vi "Get ROI Statistics String.vi"(8 "error in (no error)":errorcluster, 9 "ROI":T1, 10 "ROI Name (\"\")":string, 11 "ROI Statistics String":string) -> (0 "error out":errorcluster, 1 "Message":string)   [LabVIEW 2021, in "Image.lvlib"]
uses:
  Image.lvlib
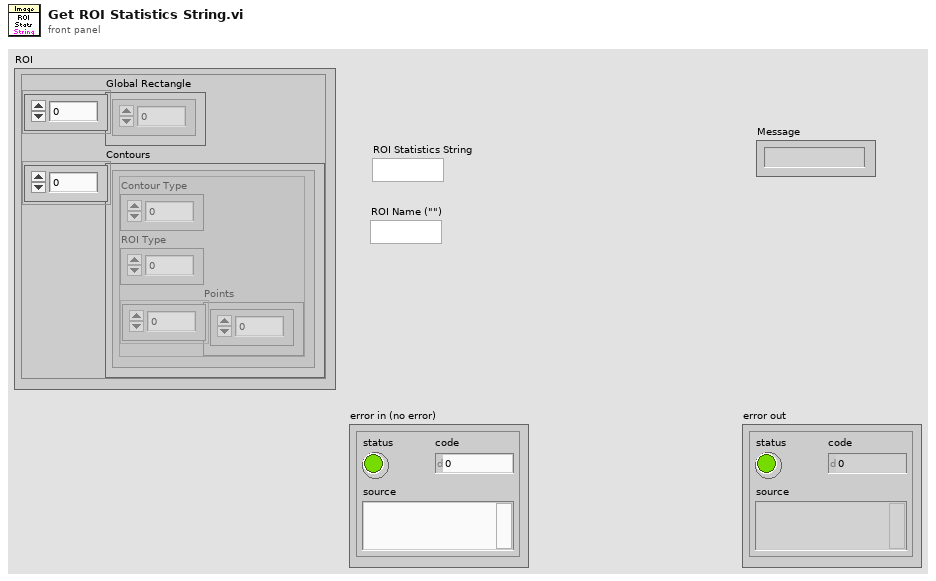
[diagram p1: front panel]
types:
  T1 = cluster{"Global Rectangle":i32[], "Contours":cluster{"Contour Type":u32, "ROI Type":u32, "Points":i32[]}[]}
  T2 = cluster{"Contour Type":u32, "ROI Type":u32, "Points":i32[]}[]
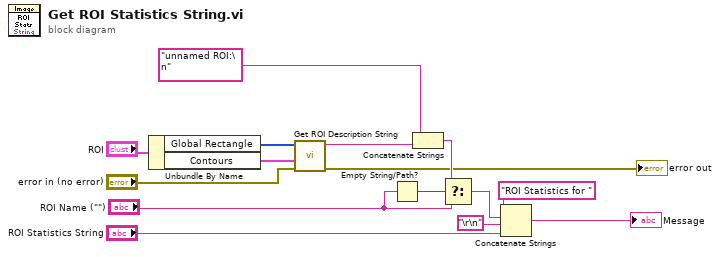
[diagram p0: block diagram]
diagram:
  n1 = Unbundle By Name("ROI") -> ("Global Rectangle"=w11:i32[], "Contours"=w10:T2)
  n2 = call "Get ROI Description String.vi"("Error In"="error in (no error)", "Contours"=w10, "Global Rectangle"=w11) -> ("Error Out"=→"error out":errorcluster, "ROI Description String"=w8:string)  [unwired: 7 in]
  n3 = Empty String/Path?(string/path="ROI Name (\"\")") -> (empty?=w13:bool)
  n4 = Concatenate Strings("unnamed ROI:\n" ("string"), w8) -> (w6:string)
  n5 = Select(t=w6, s=w13, f="ROI Name (\"\")") -> (s? t:f=w12:string)
  n6 = Concatenate Strings("ROI Statistics for " ("string"), w12, "\r\n", "ROI Statistics String") -> (→"Message":string)
